vi "dumpAccelTestData.vi"(8 "error in (no error)":errorcluster, 9 "Samples":dbl, 10 "Robot Model":T1[](array[typedef]), 11 "Communication in":refnum<class "Communication.lvclass">) -> (0 "error out":errorcluster, 2 "Mean":T1[](array[typedef]), 3 "Communication out":refnum<class "Communication.lvclass">)   [LabVIEW 2020, in "Communication.lvclass"]
uses:
  Communication.lvclass
  Controls/RobotModel.ctl
  Utilities_class/Utilities.lvclass
panel:
  out "STD":T1[](array[typedef])
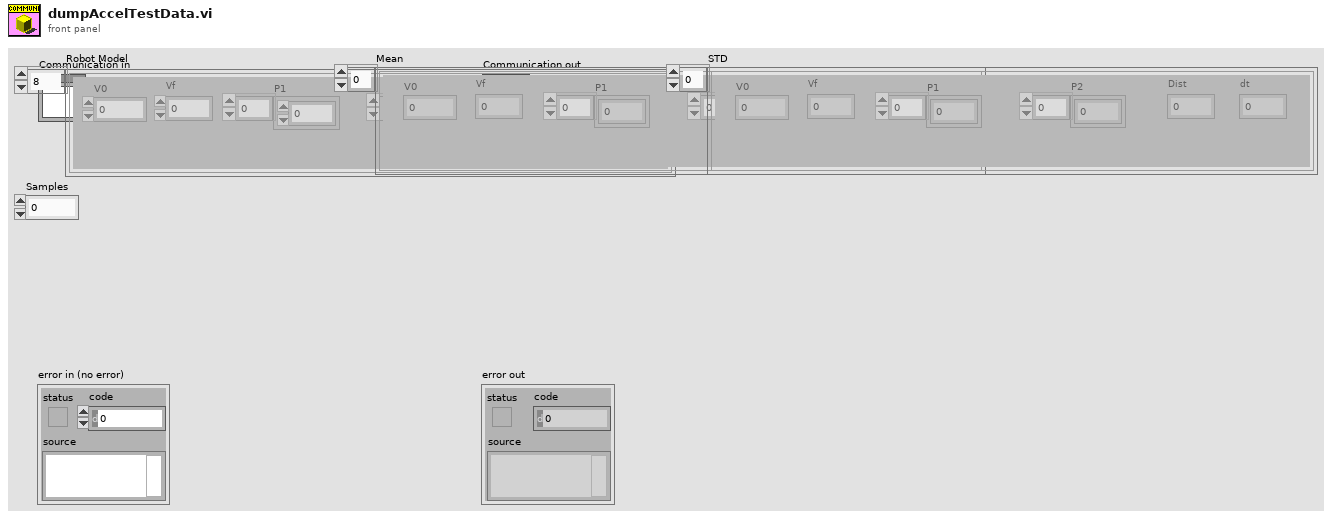
[diagram p1: front panel]
types:
  T1 = typedef "RobotModel.ctl" = cluster{"V0":dbl, "Vf":dbl, "Dist":dbl, "dt":dbl, "P1":dbl[], "P2":dbl[]}
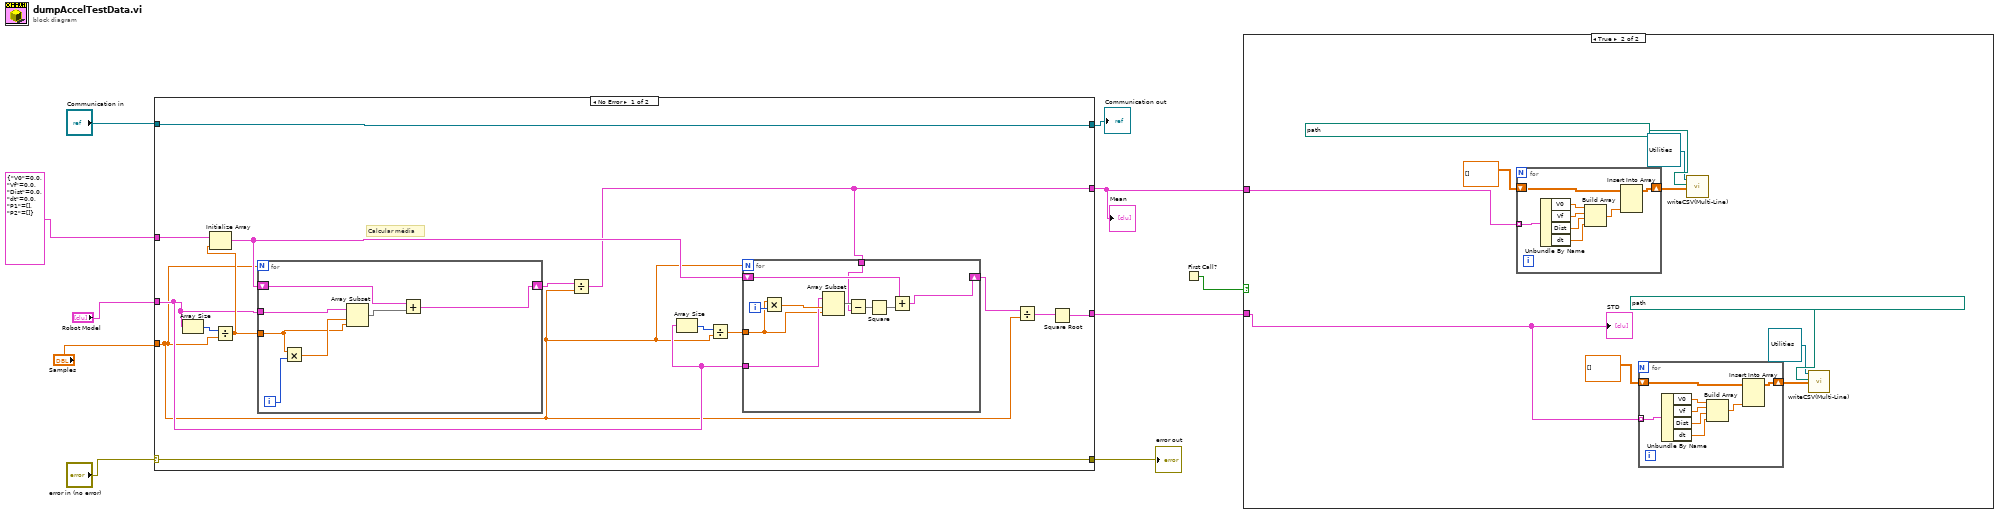
[diagram p0: block diagram]
diagram:
  n1 = case shown="No Error" "error in (no error)" {
    selector: "error in (no error)" -> [w24 w44]
    tunnel: [w24 w44] -> w9
    tunnel: [w25 w43] -> w7
    tunnel: "Communication in" -> [w25 w43]
    tunnel: "Robot Model" -> [w18 _]
    tunnel: "Samples" -> [w13 _]
    tunnel: [w15 _] -> w3
    tunnel: T1 {"V0"=0.0, "Vf"=0.0, "Dist"=0.0, "dt"=0.0, "P1"=[], "P2"=[]} ("Robot Model") -> [w21 _]
    tunnel: [w11 _] -> w2
    frame No Error {
      # "Calcular média"
      n2 = Array Size(array=w18) -> (size(s)=w23:i32)
      n3 = Divide(x=w23, y=w13) -> (x/y=w20:dbl)
      n4 = Initialize Array(w21, w20) -> (w19:T1[])
      n5 = for {
        N: w13 -> [_]
        tunnel: w18 -> [w42]
        tunnel: w20 -> [w39]
        shift-right: [w36] -> w22
        shift-left: w19 -> [w37]
        i -> [w41]
        n6 = Multiply(x=w39, y=w41) -> (x*y=w40:dbl)
        n7 = Array Subset(array=w42, index=w40, length=w39) -> (w38:T1[])
        n8 = Add(x=w37, y=w38) -> (x+y=w36:T1[])
      }
      n9 = Divide(x=w22, y=w13) -> (x/y=w15:T1[])
      n10 = Array Size(array=w18) -> (size(s)=w17:i32)
      n11 = Divide(x=w17, y=w13) -> (x/y=w16:dbl)
      n12 = for {
        N: w13 -> [_]
        tunnel: w18 -> [w32]
        tunnel: w16 -> [w30]
        shift-right: [w33] -> w14
        shift-left: w19 -> [w34]
        tunnel: w15 -> [w28]
        i -> [w31]
        n13 = Multiply(x=w30, y=w31) -> (x*y=w35:dbl)
        n14 = Array Subset(array=w32, index=w35, length=w30) -> (w29:T1[])
        n15 = Subtract(x=w29, y=w28) -> (x-y=w27:T1[])
        n16 = Square(x=w27) -> (x^2=w26:T1[])
        n17 = Add(x=w34, y=w26) -> (x+y=w33:T1[])
      }
      n18 = Divide(x=w14, y=w13) -> (x/y=w12:T1[])
      n19 = Square Root(x=w12) -> (sqrt(x)=w11:T1[])
    }
    frame Error {
    }
  }
  "error out" <- w9
  "Communication out" <- w7
  "Mean" <- w3
  n20 = First Call?() -> (First Call?: T/F=w1:bool)
  n21 = case shown="True" w1 {
    tunnel: w3 -> [_ w54]
    tunnel: w2 -> [_ w53]
    frame False {
    }
    frame True {
      n22 = for {
        tunnel: w54 -> [w70] mode=indexing
        shift-right: [w68] -> w49
        shift-left: dbl[][] [] ("Array") -> [w69]
        n23 = Unbundle By Name(w70) -> ("V0"=w67:dbl, "Vf"=w66:dbl, "Dist"=w65:dbl, "dt"=w64:dbl)
        n24 = Build Array(w67, w66, w65, w64) -> (w63:dbl[])
        n25 = Insert Into Array(array=w69, new element=w63) -> (w68:dbl[][])  [unwired: 2 in]
      }
      n26 = for {
        tunnel: w53 -> [w62] mode=indexing
        shift-right: [w60] -> w47
        shift-left: dbl[][] [] ("Array") -> [w61]
        n27 = Unbundle By Name(w62) -> ("V0"=w59:dbl, "Vf"=w58:dbl, "Dist"=w57:dbl, "dt"=w56:dbl)
        n28 = Build Array(w59, w58, w57, w56) -> (w55:dbl[])
        n29 = Insert Into Array(array=w61, new element=w55) -> (w60:dbl[][])  [unwired: 2 in]
      }
      n30 = call "writeCSV(Multi-Line).vi"("Array"=w49, "file path (use dialog)"=path "C:/Users/roboi/OneDrive/Área de Trabalho/TOIN SSL/control2021/SSL_AI/mean_values.csv", "Utilities in"=refnum<class "Utilities.lvclass"> refnum) -> ()  [unwired: 7 in, 2 out]
      n31 = call "writeCSV(Multi-Line).vi"("Array"=w47, "file path (use dialog)"=path "C:/Users/roboi/OneDrive/Área de Trabalho/TOIN SSL/control2021/SSL_AI/std_values.csv", "Utilities in"=refnum<class "Utilities.lvclass"> refnum) -> ()  [unwired: 7 in, 2 out]
      "STD" <- w53
    }
  }
